vi "OSC UDP Receiver.vi"() -> ()   [LabVIEW 2013]
doc: "This example VI shows how to read Open Sound Control (OSC) messages from UDP and dispatch them by their OSC address patterns. This VI is intended to be run with the OSC UDP Sender example VI."
uses:
  <vilib>/NIOSC/Argument to Int32 Data.vi
  <vilib>/NIOSC/Generate Error.vi
  <vilib>/NIOSC/NI_OSC.lvlib
panel:
  out "/D9":i32
  out "/D8":i32
  out "/D7":i32
  out "/D6":i32
  out "/D5":i32
  out "/D2":i32
  out "/D1":i32
  out "/D3":i32
  out "/D4":i32
  in  "stop":bool
  in  "Local Port":u16=9000
  # "Instructions:\n1. Open the sender VI (OSC UDP Sender.vi).\n2. Make sure the Remote Port in the sender VI and the Local Port in this VI are the same.\n3. Run both VIs.\n4. Change the values of the controls on the sender VI.  The indicators in this VI with the corresponding method addresses should update."
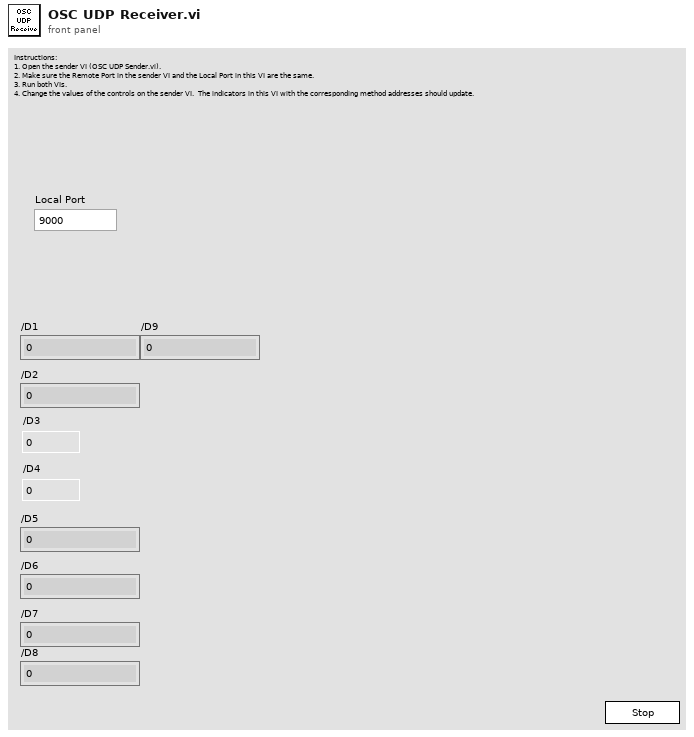
[diagram p1: front panel]
types:
  T1 = typedef "NI_OSC.lvlib/Address Space Node.ctl" = cluster{"parent index":i32, "child indexes":i32[], "address part":string, "method":bool, "data":variant}
  T2 = typedef "NI_OSC.lvlib/Method Dispatching Info.ctl" = cluster{"method address":string, "message":string, "message timetag":u64, "data":variant}
  T3 = typedef "NI_OSC.lvlib/Argument.ctl" = cluster{"argument":string, "type tag":string}
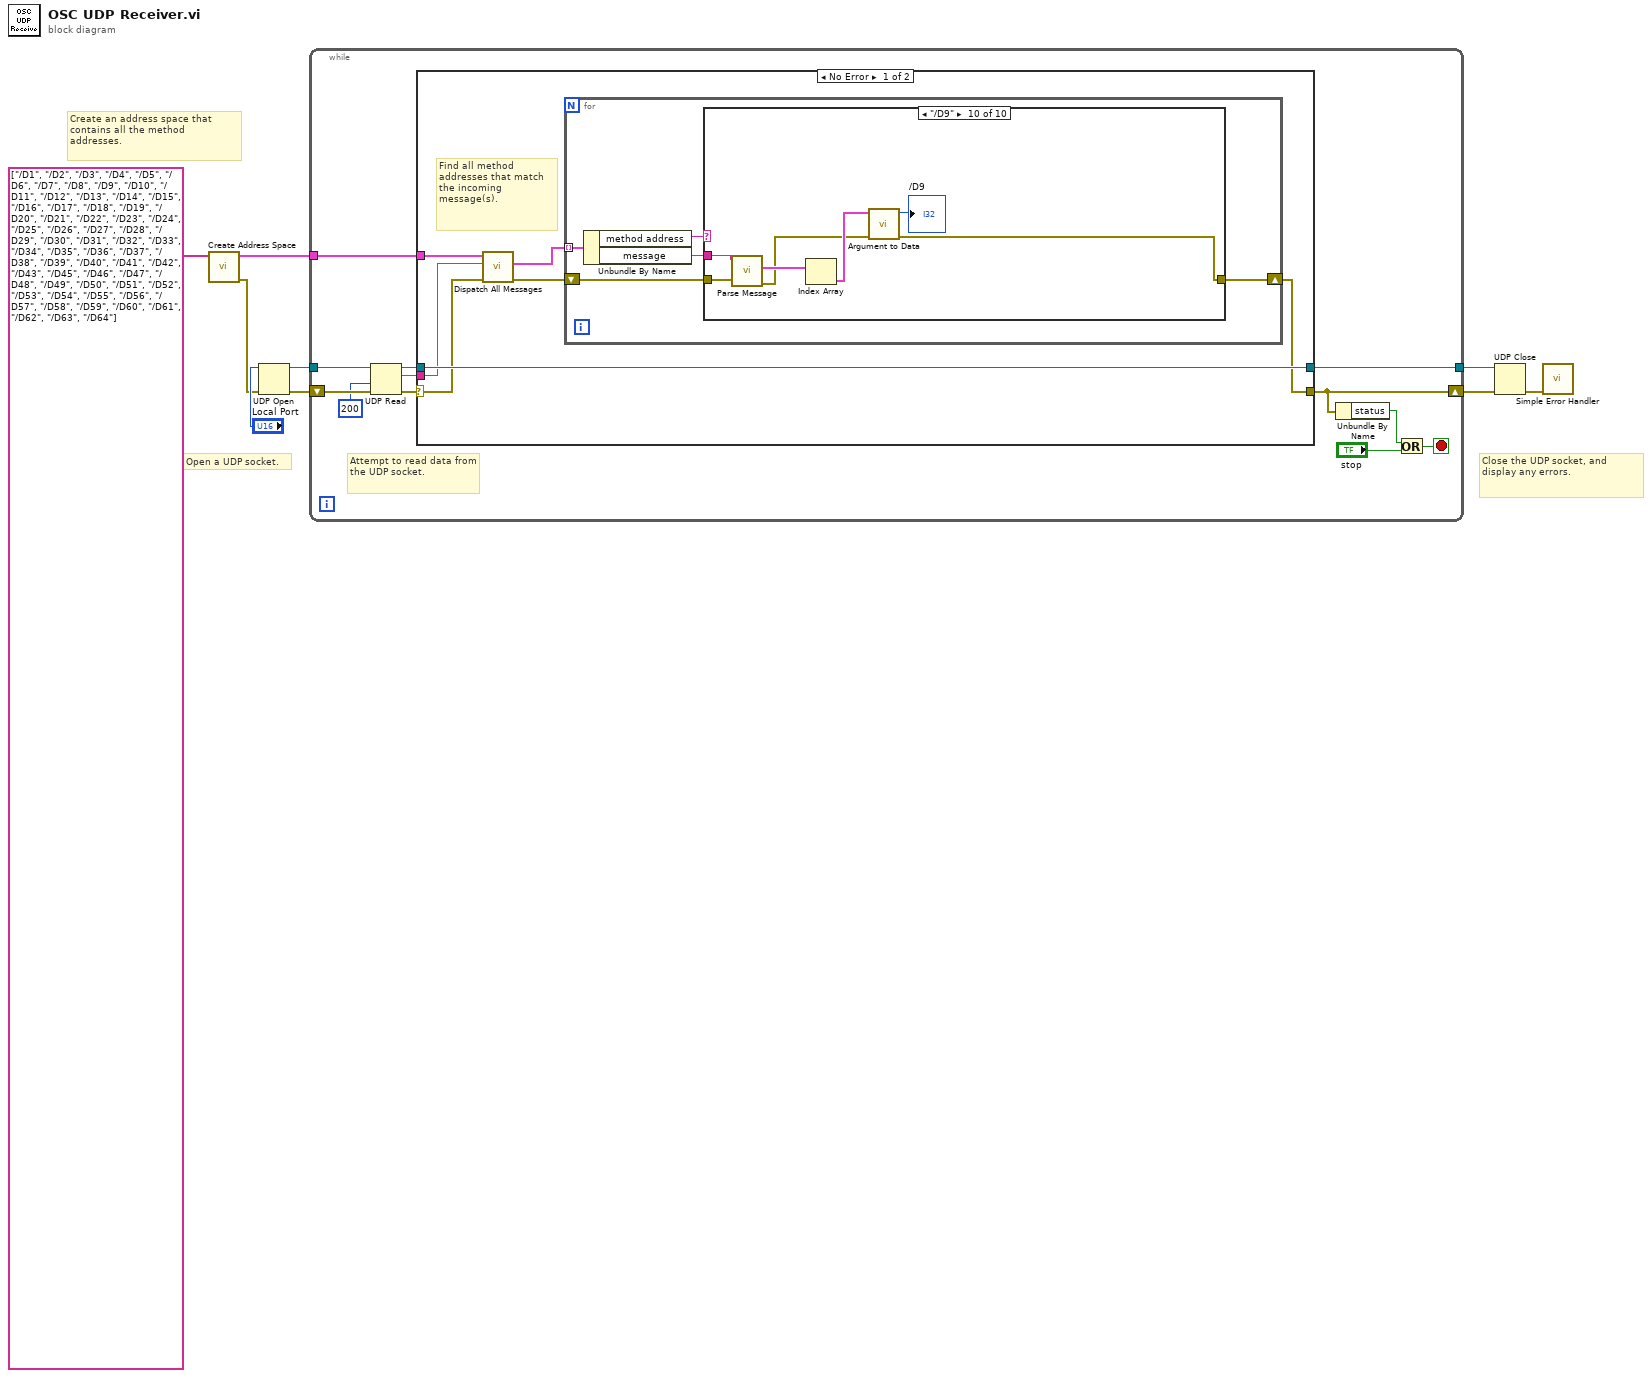
[diagram p0: block diagram]
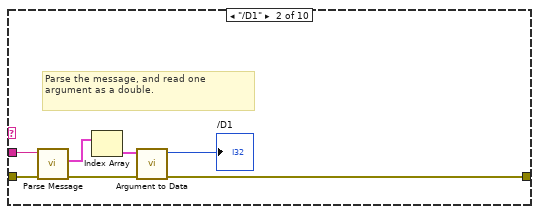
[diagram p3: hidden frame]
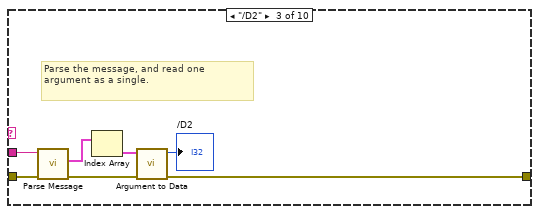
[diagram p4: hidden frame]
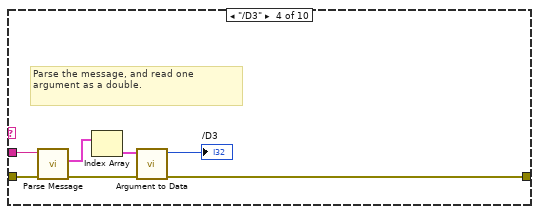
[diagram p5: hidden frame]
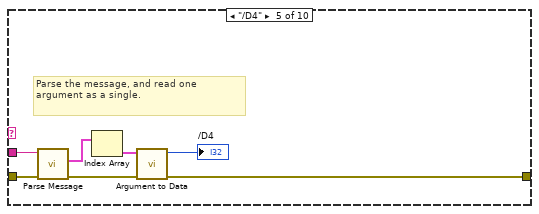
[diagram p6: hidden frame]
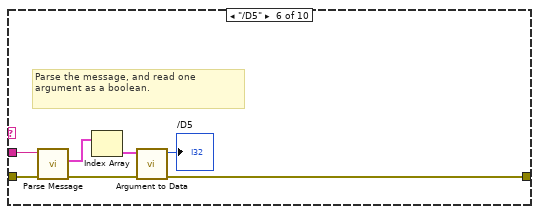
[diagram p7: hidden frame]
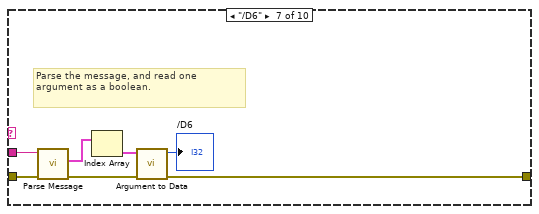
[diagram p8: hidden frame]
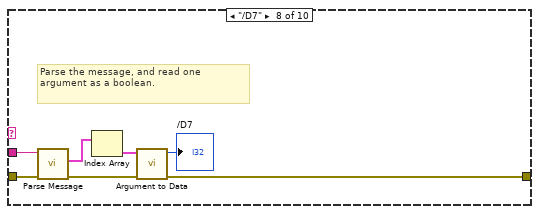
[diagram p9: hidden frame]
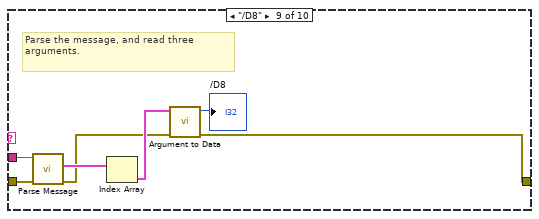
[diagram p10: hidden frame]
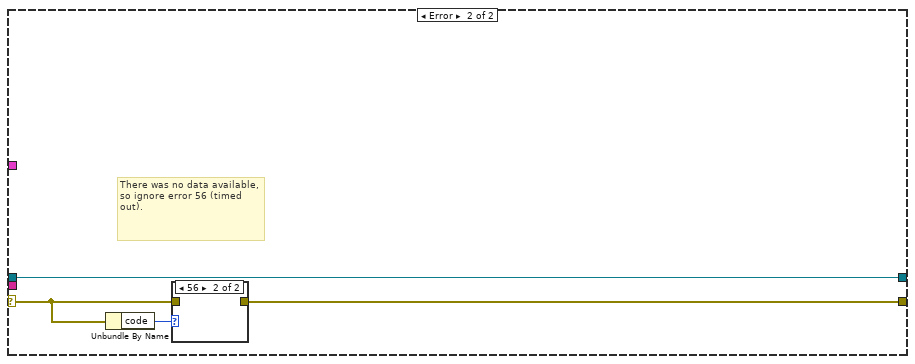
[diagram p11: hidden frame]
diagram:
  # "Close the UDP socket, and display any errors."
  # "Open a UDP socket."
  # "Create an address space that contains all the method addresses."
  n1 = call <vilib>:"Create Address Space.vi"("method addresses"=string[] ["/D1", "/D2", "/D3", "/D4", "/D5", "/D6", "/D7", "/D8", "/D9", "/D10", "/D11", "/D12", "/D13", "/D14", "/D15", "/D16", "/D17", "/D18", "/D19", "/D20", "/D21", "/D22", "/D23", "/D24", "/D25", "/D26", "/D27", "/D28", "/D29", "/D30", "/D31", "/D32", "/D33", "/D34", "/D35", "/D36", "/D37", "/D38", "/D39", "/D40", "/D41", "/D42", "/D43", "/D45", "/D46", "/D47", "/D48", "/D49", "/D50", "/D51", "/D52", "/D53", "/D54", "/D55", "/D56", "/D57", "/D58", "/D59", "/D60", "/D61", "/D62", "/D63", "/D64"]) -> ("error out"=w1:errorcluster, "address space out"=w2:T1[])  [unwired: 9 in]
  n2 = UDP Open(8:w1, 11:"Local Port") -> (port=w8:refnum<k16>, 0:w7:errorcluster)  [unwired: 3 in, 1 out]
  n3 = while {
    tunnel: w8 -> [w19]
    shift-right: [w13] -> w5
    shift-left: w7 -> [w18]
    tunnel: [w14] -> w6
    tunnel: w2 -> [w11]
    stop <- w20 stop-if-true
    # "Attempt to read data from the UDP socket."
    n4 = UDP Read(connection ID=w19, timeout ms (25000)=200, 8:w18) -> (data out=w12:string, error out=w16:errorcluster, 3:w15:refnum<k16>)  [unwired: 1 in, 2 out]
    n5 = case shown="No Error" w16 {
      selector: w16 -> [w25 w100]
      tunnel: w15 -> [w28 w98]
      tunnel: [w28 w98] -> w14
      tunnel: [w22 w99] -> w13
      tunnel: w12 -> [w27 _]
      tunnel: w11 -> [w26 _]
      frame No Error {
        # "Find all method addresses that match the incoming message(s)."
        n6 = call <vilib>:"Dispatch All Messages.vi"("error in"=w25, "packet"=w27, "address space in"=w26) -> ("error out"=w23:errorcluster, "method dispatching info"=w24:T2[])  [unwired: 6 in, 1 out]
        n7 = for {
          tunnel: w24 -> [w33] mode=indexing
          shift-right: [w31] -> w22
          shift-left: w23 -> [w32]
          n8 = Unbundle By Name(w33) -> ("method address"=w30:string, "message"=w29:string)
          n9 = case shown="\"/D9\"" w30 {
            tunnel: w32 -> [w34 w41 w48 w55 w62 w69 w76 w83 w90 w91]
            tunnel: [w34 w37 w44 w51 w58 w65 w72 w79 w85 w93] -> w31
            tunnel: w29 -> [_ w35 w43 w50 w57 w64 w71 w78 w87 w92]
            frame Default {
            }
            frame "/D1" {
              # "Parse the message, and read one argument as a double."
              n10 = call <vilib>:"Parse Message.vi"("error in"=w41, "message"=w35) -> ("error out"=w38:errorcluster, "arguments"=w40:T3[])  [unwired: 7 in, 1 out]
              n11 = Index Array(array=w40) -> (element=w39:T3)  [unwired: 1 in]
              n12 = call-poly <vilib>:"Argument to Data.vi"("error in"=w38, "int32 argument"=w39) -> ("error out"=w37:errorcluster, "int32 data"=→"/D1":i32)  [unwired: 8 in]
            }
            frame "/D2" {
              # "Parse the message, and read one argument as a single."
              n13 = call <vilib>:"Parse Message.vi"("error in"=w48, "message"=w43) -> ("error out"=w45:errorcluster, "arguments"=w47:T3[])  [unwired: 7 in, 1 out]
              n14 = Index Array(array=w47) -> (element=w46:T3)  [unwired: 1 in]
              n15 = call-poly <vilib>:"Argument to Data.vi"("error in"=w45, "int32 argument"=w46) -> ("error out"=w44:errorcluster, "int32 data"=→"/D2":i32)  [unwired: 8 in]
            }
            frame "/D3" {
              # "Parse the message, and read one argument as a double."
              n16 = call <vilib>:"Parse Message.vi"("error in"=w55, "message"=w50) -> ("error out"=w52:errorcluster, "arguments"=w54:T3[])  [unwired: 7 in, 1 out]
              n17 = Index Array(array=w54) -> (element=w53:T3)  [unwired: 1 in]
              n18 = call-poly <vilib>:"Argument to Data.vi"("error in"=w52, "int32 argument"=w53) -> ("error out"=w51:errorcluster, "int32 data"=→"/D3":i32)  [unwired: 8 in]
            }
            frame "/D4" {
              # "Parse the message, and read one argument as a single."
              n19 = call <vilib>:"Parse Message.vi"("error in"=w62, "message"=w57) -> ("error out"=w59:errorcluster, "arguments"=w61:T3[])  [unwired: 7 in, 1 out]
              n20 = Index Array(array=w61) -> (element=w60:T3)  [unwired: 1 in]
              n21 = call-poly <vilib>:"Argument to Data.vi"("error in"=w59, "int32 argument"=w60) -> ("error out"=w58:errorcluster, "int32 data"=→"/D4":i32)  [unwired: 8 in]
            }
            frame "/D5" {
              # "Parse the message, and read one argument as a boolean."
              n22 = call <vilib>:"Parse Message.vi"("error in"=w69, "message"=w64) -> ("error out"=w66:errorcluster, "arguments"=w68:T3[])  [unwired: 7 in, 1 out]
              n23 = Index Array(array=w68) -> (element=w67:T3)  [unwired: 1 in]
              n24 = call-poly <vilib>:"Argument to Data.vi"("error in"=w66, "int32 argument"=w67) -> ("error out"=w65:errorcluster, "int32 data"=→"/D5":i32)  [unwired: 8 in]
            }
            frame "/D6" {
              # "Parse the message, and read one argument as a boolean."
              n25 = call <vilib>:"Parse Message.vi"("error in"=w76, "message"=w71) -> ("error out"=w73:errorcluster, "arguments"=w75:T3[])  [unwired: 7 in, 1 out]
              n26 = Index Array(array=w75) -> (element=w74:T3)  [unwired: 1 in]
              n27 = call-poly <vilib>:"Argument to Data.vi"("error in"=w73, "int32 argument"=w74) -> ("error out"=w72:errorcluster, "int32 data"=→"/D6":i32)  [unwired: 8 in]
            }
            frame "/D7" {
              # "Parse the message, and read one argument as a boolean."
              n28 = call <vilib>:"Parse Message.vi"("error in"=w83, "message"=w78) -> ("error out"=w80:errorcluster, "arguments"=w82:T3[])  [unwired: 7 in, 1 out]
              n29 = Index Array(array=w82) -> (element=w81:T3)  [unwired: 1 in]
              n30 = call-poly <vilib>:"Argument to Data.vi"("error in"=w80, "int32 argument"=w81) -> ("error out"=w79:errorcluster, "int32 data"=→"/D7":i32)  [unwired: 8 in]
            }
            frame "/D8" {
              # "Parse the message, and read three arguments."
              n31 = call <vilib>:"Parse Message.vi"("error in"=w90, "message"=w87) -> ("error out"=w86:errorcluster, "arguments"=w89:T3[])  [unwired: 7 in, 1 out]
              n32 = Index Array(array=w89) -> (element=w88:T3)  [unwired: 1 in]
              n33 = call-poly <vilib>:"Argument to Data.vi"("error in"=w86, "int32 argument"=w88) -> ("error out"=w85:errorcluster, "int32 data"=→"/D8":i32)  [unwired: 8 in]
            }
            frame "/D9" {
              n34 = call <vilib>:"Parse Message.vi"("error in"=w91, "message"=w92) -> ("error out"=w95:errorcluster, "arguments"=w97:T3[])  [unwired: 7 in, 1 out]
              n35 = Index Array(array=w97) -> (element=w96:T3)  [unwired: 1 in]
              n36 = call-poly <vilib>:"Argument to Data.vi"("error in"=w95, "int32 argument"=w96) -> ("error out"=w93:errorcluster, "int32 data"=→"/D9":i32)  [unwired: 8 in]
            }
          }
        }
      }
      frame Error {
        # "There was no data available, so ignore error 56 (timed out)."
        n37 = Unbundle By Name(w100) -> ("code"=w101:i32)
        n38 = case shown="56" w101 {
          tunnel: w100 -> [w102 _]
          tunnel: [w102 _] -> w99
          frame Default {
          }
          frame 56 {
          }
        }
      }
    }
    n39 = Unbundle By Name(w13) -> ("status"=w21:bool)
    n40 = Or(x=w21, y="stop") -> (x .or. y?=w20:bool)
  }
  n41 = UDP Close(connection ID=w6, 8:w5) -> (error out=w4:errorcluster)  [unwired: 1 out]
  n42 = call <vilib>:"Simple Error Handler.vi"("error in (no error)"=w4) -> ()  [unwired: 4 in, 5 out]
